vi "Disable.vi"(11 "logger in":refnum<class "Logger.lvclass">) -> (3 "logger out":refnum<class "Logger.lvclass">)   [LabVIEW 2018, in "Logging.lvlib" / "Logger.lvclass"]
uses:
  Logger.lvclass
  Logger.lvclass/Logger.ctl
panel:
  # "Connector Pane"
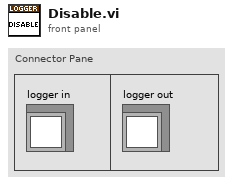
[diagram p1: front panel]
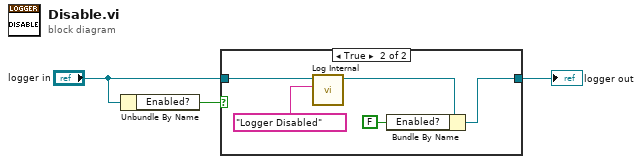
[diagram p0: block diagram]
diagram:
  n1 = Unbundle By Name("logger in") -> ("Enabled?"=w1:bool)
  n2 = case shown="True" w1 {
    tunnel: "logger in" -> [w4 w7]
    tunnel: [w4 w5] -> w3
    frame False {
    }
    frame True {
      n3 = call "Log Internal.vi"("message"="Logger Disabled", "logger in"=w7) -> ("logger out"=w6:refnum<class "Logger.lvclass">)  [unwired: 9 in]
      n4 = Bundle By Name(cluster=w6, "Enabled?"=FALSE) -> (w5:refnum<class "Logger.lvclass">)
    }
  }
  "logger out" <- w3
